vi "alarm output.vi"(8 "error in (no error)":errorcluster caption="错误输入（无错误）", 11 "采配水V3告警 输入":refnum<class "采配水V3告警.lvclass">) -> (0 "error out":errorcluster caption="错误输出", 2 "output":cluster{"code":i32, "msg":string}[](array[cluster]), 3 "采配水V3告警 输出":refnum<class "采配水V3告警.lvclass">)   [LabVIEW 2016, in "PLC.lvlib" / "采配水V3告警.lvclass"]
uses:
  PLC.lvlib
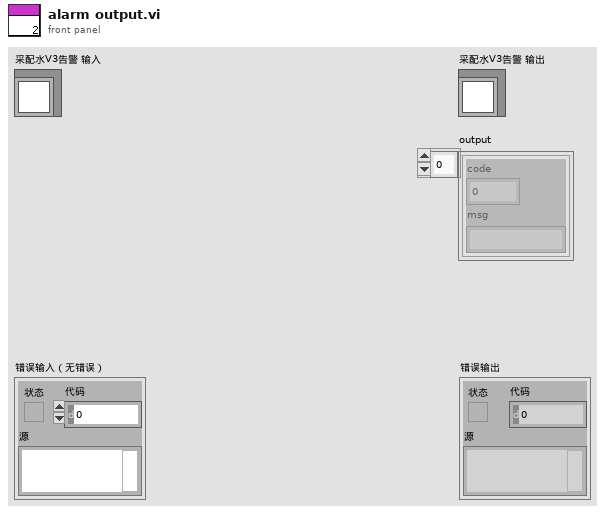
[diagram p1: front panel]
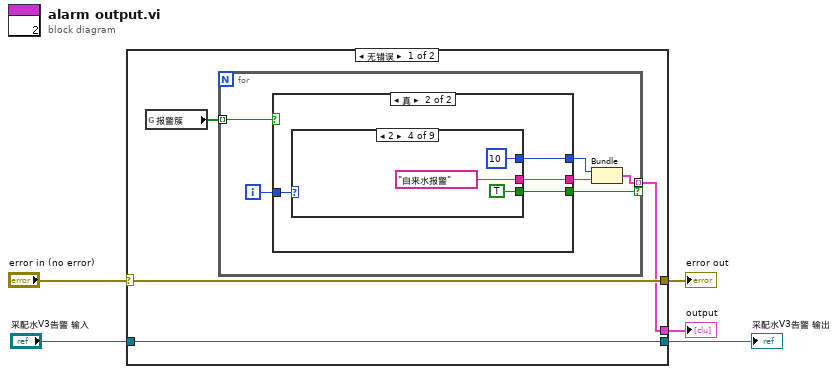
[diagram p0: block diagram]
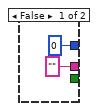
[diagram p2: hidden frame]
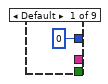
[diagram p3: hidden frame]
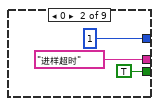
[diagram p4: hidden frame]
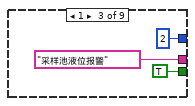
[diagram p5: hidden frame]
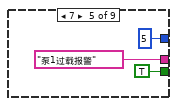
[diagram p6: hidden frame]
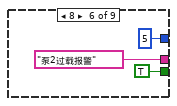
[diagram p7: hidden frame]
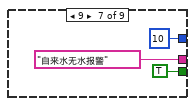
[diagram p8: hidden frame]
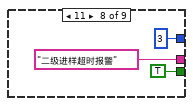
[diagram p9: hidden frame]
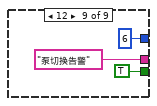
[diagram p10: hidden frame]
diagram:
  n1 = case shown="无错误" "error in (no error)" {
    selector: "error in (no error)" -> [w8 w48]
    tunnel: [w8 w48] -> w4
    tunnel: [w6 _] -> w3
    tunnel: "采配水V3告警 输入" -> [w7 w47]
    tunnel: [w7 w47] -> w2
    frame No Error {
      n2 = global read "采配水全局变量.vi" "报警簇"() -> (w9:bool[])
      n3 = for {
        tunnel: w9 -> [w15] mode=indexing
        tunnel: [w11] -> w6 mode=indexing if=w14
        i -> [w12]
        n4 = case shown="真" w15 {
          tunnel: w12 -> [_ w19]
          tunnel: ["" w21] -> w13
          tunnel: [_ w20] -> w14
          tunnel: [0 w18] -> w10
          frame False {
          }
          frame True {
            n5 = case shown="2" w19 {
              tunnel: [_ "进样超时" ("组合框") "采样池液位报警" ("组合框") "自来水报警" ("组合框") "泵1过载报警" ("组合框") "泵2过载报警" ("组合框") "自来水无水报警" ("组合框") "二级进样超时报警" ("组合框") "泵切换告警" ("组合框")] -> w21
              tunnel: [_ TRUE TRUE TRUE TRUE TRUE TRUE TRUE TRUE] -> w20
              tunnel: [0 1 2 10 5 5 10 3 6] -> w18
              frame Default {
              }
              frame 0 {
              }
              frame 1 {
              }
              frame 2 {
              }
              frame 7 {
              }
              frame 8 {
              }
              frame 9 {
              }
              frame 11 {
              }
              frame 12 {
              }
            }
          }
        }
        n6 = Bundle(w10, "组合框"=w13) -> (w11:cluster{i32, "组合框":string})  [unwired: 1 in]
      }
    }
    frame Error {
    }
  }
  "error out" <- w4
  "采配水V3告警 输出" <- w2
  "output" <- w3
